vi "ConvertData.vi"(8 "error in (no error)":errorcluster, 11 "recordset data":variant[][](array[variant])) -> (0 "error out":errorcluster, 3 "SR List":T1[](array[typedef]) {"SR#" format="%#_10g"})   [LabVIEW 2017, in "Server.lvlib" / "Oracle.lvlib"]
doc: "Converts the 2D-Variant-Array from the Database Query to the SR List.ctl Array of Clusters for further processing."
uses:
  Oracle.lvlib
  TypeDefs/SR Data.ctl
  <vilib>/addons/database/_DB Variant To Data/Database Variant To Data.xnode
  Server.lvlib
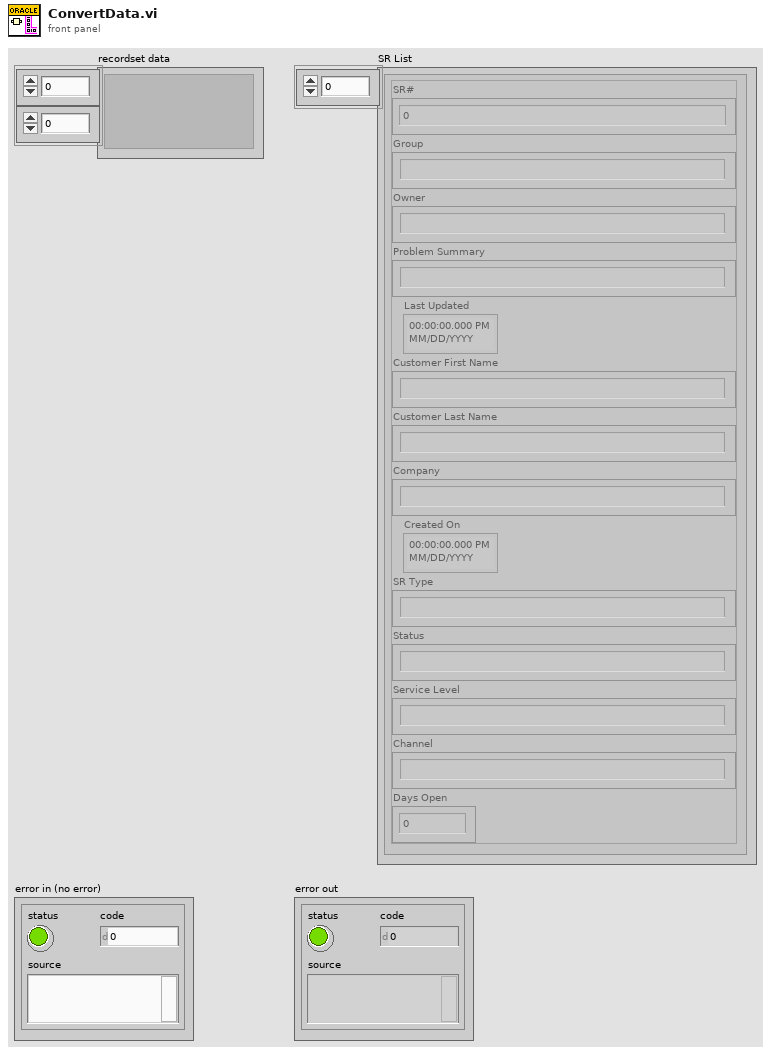
[diagram p1: front panel]
types:
  T1 = typedef "Server.lvlib/SR Data.ctl" = cluster{"SR#":dbl, "Group":string, "Owner":string, "Problem Summary":string, "Last Updated":timestamp, "Customer First Name":string, "Customer Last Name":string, "Company":string, "Created On":timestamp, "SR Type":string, "Status":string, "Service Level":string, "Channel":string, "Days Open":dbl}
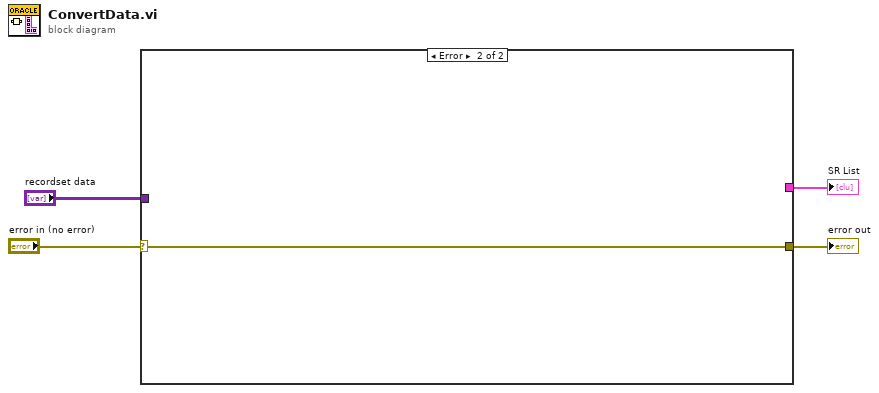
[diagram p0: block diagram]
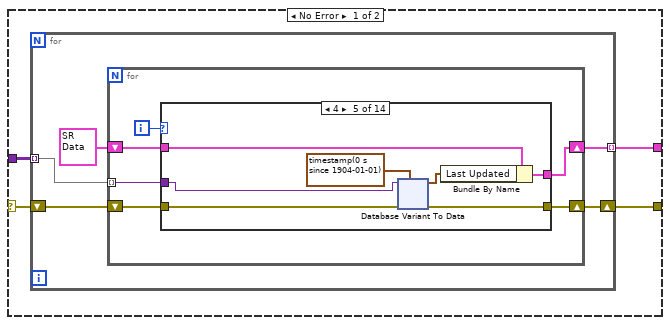
[diagram p2: hidden frame]
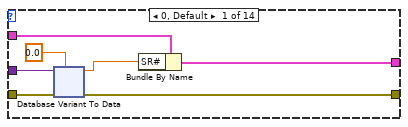
[diagram p3: hidden frame]
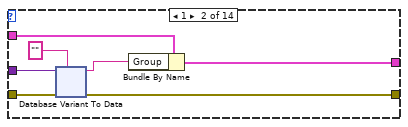
[diagram p4: hidden frame]
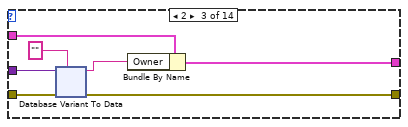
[diagram p5: hidden frame]
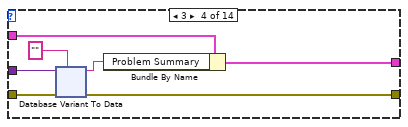
[diagram p6: hidden frame]
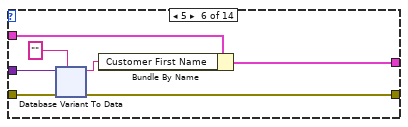
[diagram p7: hidden frame]
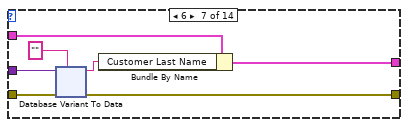
[diagram p8: hidden frame]
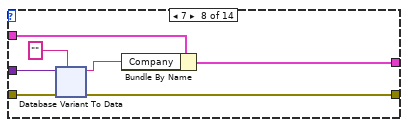
[diagram p9: hidden frame]
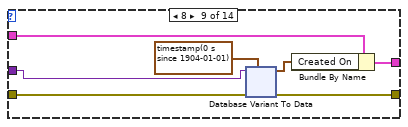
[diagram p10: hidden frame]
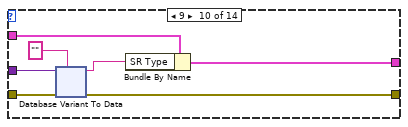
[diagram p11: hidden frame]
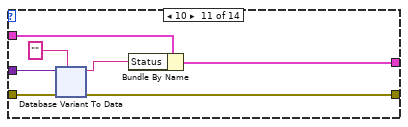
[diagram p12: hidden frame]
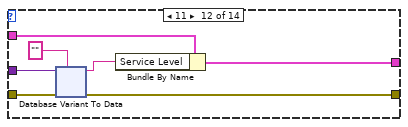
[diagram p13: hidden frame]
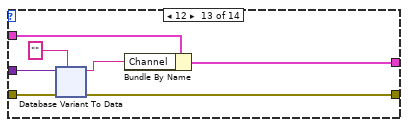
[diagram p14: hidden frame]
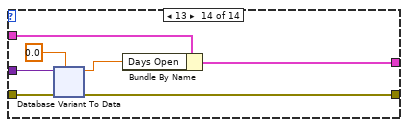
[diagram p15: hidden frame]
diagram:
  n1 = case shown="Error" "error in (no error)" {
    selector: "error in (no error)" -> [w5 w592]
    tunnel: [w8 w592] -> w4
    tunnel: "recordset data" -> [w7 _]
    tunnel: [w6 _] -> w2
    frame No Error {
      n2 = for {
        tunnel: w7 -> [w13] mode=indexing
        tunnel: [w12] -> w6 mode=indexing
        shift-right: [w9] -> w8
        shift-left: w5 -> [w10]
        n3 = for {
          tunnel: w13 -> [w18] mode=indexing
          shift-right: [w16] -> w12
          shift-left: T1 {"SR#"=0.0, "Group"="", "Owner"="", "Problem Summary"="", "Last Updated"=timestamp(0 s since 1904-01-01), "Customer First Name"="", "Customer Last Name"="", "Company"="", "Created On"=timestamp(0 s since 1904-01-01), "SR Type"="", "Status"="", "Service Level"="", "Channel"="", "Days Open"=0.0} ("SR Data") -> [w17]
          shift-right: [w14] -> w9
          shift-left: w10 -> [w15]
          i -> [w19]
          n4 = case shown="4" w19 {
            tunnel: w18 -> [w24 w64 w103 w142 w182 w233 w272 w311 w351 w402 w441 w480 w519 w557]
            tunnel: w17 -> [w26 w63 w102 w141 w180 w232 w271 w310 w349 w401 w440 w479 w518 w559]
            tunnel: [w22 w61 w100 w139 w179 w230 w269 w308 w348 w399 w438 w477 w516 w555] -> w16
            tunnel: w15 -> [w21 w60 w99 w138 w177 w229 w268 w307 w346 w398 w437 w476 w515 w554]
            tunnel: [w20 w59 w98 w137 w176 w228 w267 w306 w345 w397 w436 w475 w514 w553] -> w14
            frame 0, Default {
              n5 = xnode "Database Variant To Data"("database variant"=w24, "error in (no error)"=w21, "type"=0.0) -> ("data"=w23:dbl, "error out"=w20:errorcluster)
              n6 = Bundle By Name(cluster=w26, "SR#"=w23) -> (w22:T1)
            }
            frame 1 {
              n7 = xnode "Database Variant To Data"("database variant"=w64, "error in (no error)"=w60, "type"="" ("String")) -> ("data"=w62:string, "error out"=w59:errorcluster)
              n8 = Bundle By Name(cluster=w63, "Group"=w62) -> (w61:T1)
            }
            frame 2 {
              n9 = xnode "Database Variant To Data"("database variant"=w103, "error in (no error)"=w99, "type"="" ("String")) -> ("data"=w101:string, "error out"=w98:errorcluster)
              n10 = Bundle By Name(cluster=w102, "Owner"=w101) -> (w100:T1)
            }
            frame 3 {
              n11 = xnode "Database Variant To Data"("database variant"=w142, "error in (no error)"=w138, "type"="" ("String")) -> ("data"=w140:string, "error out"=w137:errorcluster)
              n12 = Bundle By Name(cluster=w141, "Problem Summary"=w140) -> (w139:T1)
            }
            frame 4 {
              n13 = xnode "Database Variant To Data"("database variant"=w182, "error in (no error)"=w177, "type"=timestamp(0 s since 1904-01-01)) -> ("data"=w178:timestamp, "error out"=w176:errorcluster)
              n14 = Bundle By Name(cluster=w180, "Last Updated"=w178) -> (w179:T1)
            }
            frame 5 {
              n15 = xnode "Database Variant To Data"("database variant"=w233, "error in (no error)"=w229, "type"="" ("String")) -> ("data"=w231:string, "error out"=w228:errorcluster)
              n16 = Bundle By Name(cluster=w232, "Customer First Name"=w231) -> (w230:T1)
            }
            frame 6 {
              n17 = xnode "Database Variant To Data"("database variant"=w272, "error in (no error)"=w268, "type"="" ("String")) -> ("data"=w270:string, "error out"=w267:errorcluster)
              n18 = Bundle By Name(cluster=w271, "Customer Last Name"=w270) -> (w269:T1)
            }
            frame 7 {
              n19 = xnode "Database Variant To Data"("database variant"=w311, "error in (no error)"=w307, "type"="" ("String")) -> ("data"=w309:string, "error out"=w306:errorcluster)
              n20 = Bundle By Name(cluster=w310, "Company"=w309) -> (w308:T1)
            }
            frame 8 {
              n21 = xnode "Database Variant To Data"("database variant"=w351, "error in (no error)"=w346, "type"=timestamp(0 s since 1904-01-01)) -> ("data"=w347:timestamp, "error out"=w345:errorcluster)
              n22 = Bundle By Name(cluster=w349, "Created On"=w347) -> (w348:T1)
            }
            frame 9 {
              n23 = xnode "Database Variant To Data"("database variant"=w402, "error in (no error)"=w398, "type"="" ("String")) -> ("data"=w400:string, "error out"=w397:errorcluster)
              n24 = Bundle By Name(cluster=w401, "SR Type"=w400) -> (w399:T1)
            }
            frame 10 {
              n25 = xnode "Database Variant To Data"("database variant"=w441, "error in (no error)"=w437, "type"="" ("String")) -> ("data"=w439:string, "error out"=w436:errorcluster)
              n26 = Bundle By Name(cluster=w440, "Status"=w439) -> (w438:T1)
            }
            frame 11 {
              n27 = xnode "Database Variant To Data"("database variant"=w480, "error in (no error)"=w476, "type"="" ("String")) -> ("data"=w478:string, "error out"=w475:errorcluster)
              n28 = Bundle By Name(cluster=w479, "Service Level"=w478) -> (w477:T1)
            }
            frame 12 {
              n29 = xnode "Database Variant To Data"("database variant"=w519, "error in (no error)"=w515, "type"="" ("String")) -> ("data"=w517:string, "error out"=w514:errorcluster)
              n30 = Bundle By Name(cluster=w518, "Channel"=w517) -> (w516:T1)
            }
            frame 13 {
              n31 = xnode "Database Variant To Data"("database variant"=w557, "error in (no error)"=w554, "type"=0.0) -> ("data"=w556:dbl, "error out"=w553:errorcluster)
              n32 = Bundle By Name(cluster=w559, "Days Open"=w556) -> (w555:T1)
            }
          }
        }
      }
    }
    frame Error {
    }
  }
  "error out" <- w4
  "SR List" <- w2
